vi "programa2velocimetrocu.vi"() -> ()   [LabVIEW 2011]
panel:
  out "Rango":string
  out "121-180":bool
  out "81-120":bool
  out "1-80":bool
  out "Velocidad":i32(knob) scale=0.0..180.0
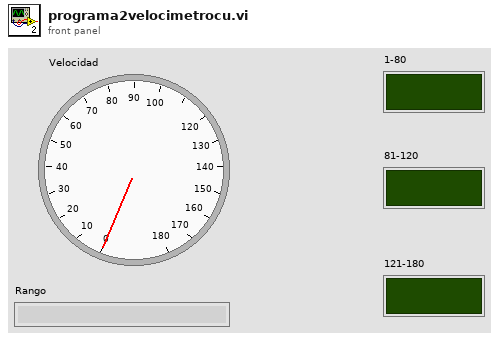
[diagram p1: front panel]
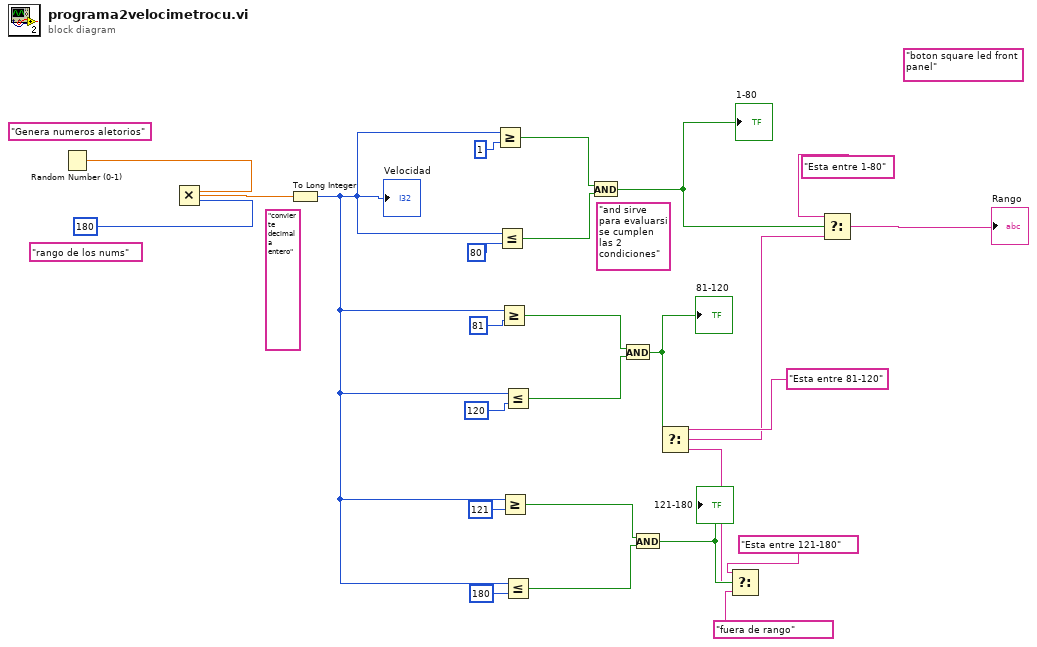
[diagram p0: block diagram]
diagram:
  (unwired) "boton square led front panel"
  (unwired) "and sirve para evaluarsi se cumplen las 2 condiciones"
  (unwired) "rango de los nums"
  (unwired) "convierte decimal a entero"
  (unwired) "Genera numeros aletorios"
  n1 = Random Number (0-1)() -> (number: 0 to 1=w26:dbl)
  n2 = Multiply(x=w26, y=180) -> (x*y=w24:dbl)
  n3 = To Long Integer(number=w24) -> (32bit integer=w15:i32)
  "Velocidad" <- w15
  n4 = Greater Or Equal?(x=w15, y=1) -> (x >= y?=w21:bool)
  n5 = Less Or Equal?(x=w15, y=80) -> (x <= y?=w20:bool)
  n6 = Greater Or Equal?(x=w15, y=81) -> (x >= y?=w12:bool)
  n7 = Greater Or Equal?(x=w15, y=121) -> (x >= y?=w14:bool)
  n8 = Less Or Equal?(x=w15, y=120) -> (x <= y?=w11:bool)
  n9 = Less Or Equal?(x=w15, y=180) -> (x <= y?=w13:bool)
  n10 = And(x=w21, y=w20) -> (x .and. y?=w10:bool)
  "1-80" <- w10
  n11 = And(x=w12, y=w11) -> (x .and. y?=w7:bool)
  "81-120" <- w7
  n12 = And(x=w14, y=w13) -> (x .and. y?=w2:bool)
  "121-180" <- w2
  n13 = Select(t="Esta entre 121-180", s=w2, f="fuera de rango") -> (s? t:f=w1:string)
  n14 = Select(t="Esta entre 81-120", s=w7, f=w1) -> (s? t:f=w5:string)
  n15 = Select(t="Esta entre 1-80", s=w10, f=w5) -> (s? t:f=→"Rango":string)
